vi "distance.vi"() -> ()   [LabVIEW 2014]
panel:
  out "两点间距离":dbl
  in  "第二个点Y":dbl
  in  "第二个点X":dbl
  in  "第一个点Y":dbl
  in  "第一个点X":dbl
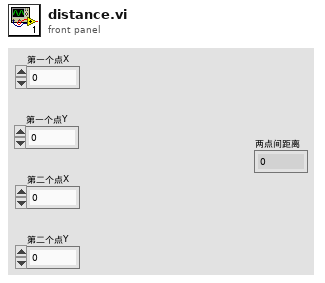
[diagram p1: front panel]
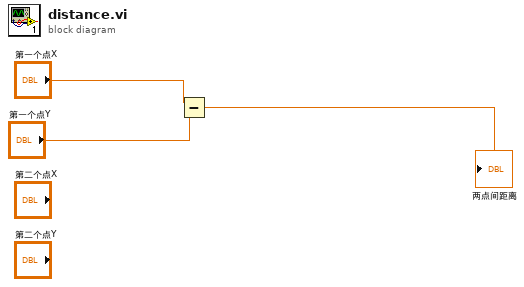
[diagram p0: block diagram]
diagram:
  n1 = Subtract(x="第一个点X", y="第一个点Y") -> (x-y=→"两点间距离":dbl)
